vi "Input Entry Input Type Change.vi"(8 "Input":T2, 10 "Refnums":T1, 11 "Input Control Refnum":refnum<vi>) -> (3 "Input Control Refnum out":refnum<vi>)   [LabVIEW 2015, in "CallVIStep.lvclass"]
uses:
  CallVIStep.lvclass
  VI Input Control Typedef.ctl
  VI Input Type Typedef.ctl
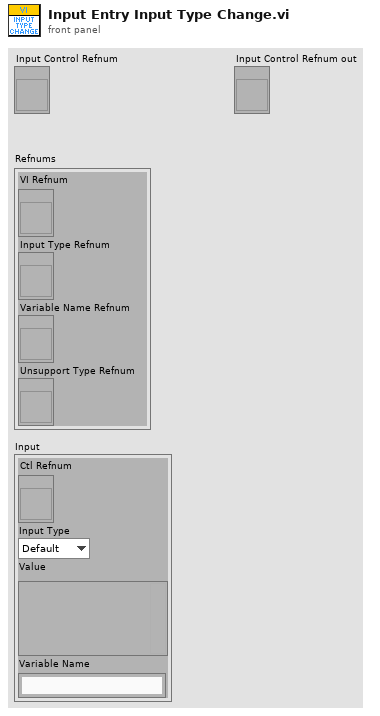
[diagram p1: front panel]
types:
  T1 = cluster{"VI Refnum":refnum<vi>, "Input Type Refnum":refnum<vi>, "Variable Name Refnum":refnum<vi>, "Unsupport Type Refnum":refnum<vi>}
  T2 = typedef "CallVIStep.lvclass/VI Input Control Typedef.ctl" = cluster{"Ctl Refnum":refnum<vi>, "Input Type":T3, "Value":variant, "Variable Name":string}
  T3 = typedef "CallVIStep.lvclass/VI Input Type Typedef.ctl" = enum16{"Default", "Value", "Variable"}
  T4 = enum8{"Enabled", "Disabled", "Disabled and Grayed Out"}
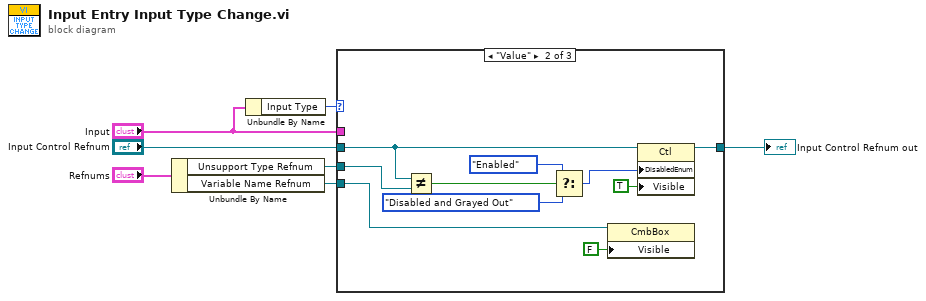
[diagram p0: block diagram]
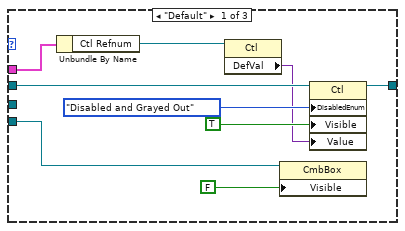
[diagram p2: hidden frame]
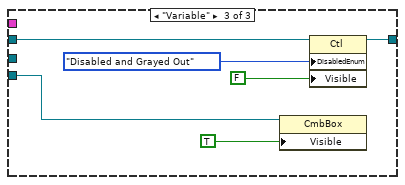
[diagram p3: hidden frame]
diagram:
  n1 = Unbundle By Name("Refnums") -> ("Unsupport Type Refnum"=w2:refnum<vi>, "Variable Name Refnum"=w1:refnum<vi>)
  n2 = Unbundle By Name("Input") -> ("Input Type"=w4:T3)
  n3 = case shown="\"Value\"" w4 {
    tunnel: "Input Control Refnum" -> [w16 w22 w32]
    tunnel: [w15 w26 w31] -> w6
    tunnel: "Input" -> [w14 _ _]
    tunnel: w1 -> [w12 w24 w28]
    tunnel: w2 -> [_ w21 _]
    frame "Default" {
      n4 = Unbundle By Name(w14) -> ("Ctl Refnum"=w13:refnum<vi>)
      n5 = property class="Ctl"(reference=w13) -> ("DefVal"=w8:variant)  [unwired: 1 in, 2 out]
      n6 = property class="CmbBox"(reference=w12, "Visible"=FALSE) -> ()  [unwired: 1 in, 2 out]
      n7 = property class="Ctl"(reference=w16, "DisabledEnum"=T4."Disabled and Grayed Out" ("Disabled"), "Visible"=TRUE, "Value"=w8) -> (reference out=w15:refnum<vi>)  [unwired: 1 in, 1 out]
    }
    frame "Value" {
      n8 = Not Equal?(x=w22, y=w21) -> (x != y?=w18:bool)
      n9 = Select(t=T4."Enabled" ("Disabled"), s=w18, f=T4."Disabled and Grayed Out" ("Disabled")) -> (s? t:f=w17:T4)
      n10 = property class="CmbBox"(reference=w24, "Visible"=FALSE) -> ()  [unwired: 1 in, 2 out]
      n11 = property class="Ctl"(reference=w22, "DisabledEnum"=w17, "Visible"=TRUE) -> (reference out=w26:refnum<vi>)  [unwired: 1 in, 1 out]
    }
    frame "Variable" {
      n12 = property class="CmbBox"(reference=w28, "Visible"=TRUE) -> ()  [unwired: 1 in, 2 out]
      n13 = property class="Ctl"(reference=w32, "DisabledEnum"=T4."Disabled and Grayed Out" ("Disabled"), "Visible"=FALSE) -> (reference out=w31:refnum<vi>)  [unwired: 1 in, 1 out]
    }
  }
  "Input Control Refnum out" <- w6
